vi "RTM CreateFramesSubSection.vi"(8 "error in (no error)":errorcluster, 11 "Node Ptr":T1 format="%.0x") -> (0 "error out":errorcluster, 3 "Node Ptr 2":T1 format="%.0x")   [LabVIEW 2018, in "CAN Gateway System Explorer.lvlib"]
uses:
  CAN Gateway System Explorer.lvlib
  <vilib>/NI Veristand/Custom Device API/Custom Device Item Ref.ctl
  <vilib>/NI Veristand/Custom Device API/Custom Device Channel.ctl
  <vilib>/NI Veristand/Custom Device API/Custom Device Channel Type.ctl
  Shared/Constants.vi
  <vilib>/NI Veristand/Custom Device API/Custom Device API.lvlib
  Shared/CAN Gateway Shared.lvlib
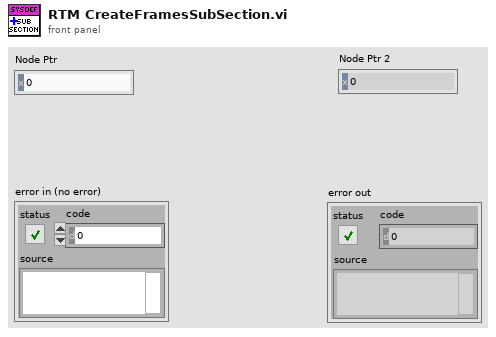
[diagram p1: front panel]
types:
  T1 = typedef "Custom Device API.lvlib/Custom Device Item Ref.ctl" = u64
  T2 = typedef "Custom Device API.lvlib/Custom Device Channel.ctl" = cluster{"Type":T3, "Units":string, "Default Value":dbl, "Faultable":bool, "Scalable":bool}
  T3 = typedef "Custom Device API.lvlib/Custom Device Channel Type.ctl" = enum16{"Input", "Output"}
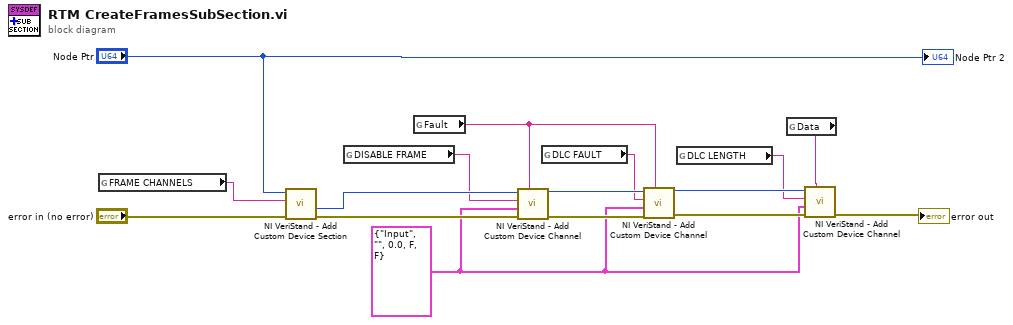
[diagram p0: block diagram]
diagram:
  w4 = T2 {"Type"=enum."Input", "Units"="", "Default Value"=0.0, "Faultable"=FALSE, "Scalable"=FALSE} ("Channel")
  n1 = global read "Constants.vi" "FRAME CHANNELS"() -> (w14:string)
  n2 = call <vilib>:"NI VeriStand - Add Custom Device Section.vi"("error in (no error)"="error in (no error)", "Section Name"=w14, "Parent Ref in"="Node Ptr") -> ("error out"=w12:errorcluster, "Section Ptr"=w13:T1)  [unwired: 5 in, 2 out]
  n3 = global read "Constants.vi" "DISABLE FRAME"() -> (w11:string)
  n4 = global read "Constants.vi" "Fault"() -> (w3:string)
  n5 = call <vilib>:"NI VeriStand - Add Custom Device Channel.vi"("GUID (Default Channel)"=w3, "error in (no error)"=w12, "Channel"=w4, "Channel Name"=w11, "Parent Ref in"=w13) -> ("error out"=w8:errorcluster, "Parent Ref out"=w10:T1)  [unwired: 3 in, 2 out]
  n6 = global read "Constants.vi" "DLC FAULT"() -> (w9:string)
  n7 = call <vilib>:"NI VeriStand - Add Custom Device Channel.vi"("GUID (Default Channel)"=w3, "error in (no error)"=w8, "Channel"=w4, "Channel Name"=w9, "Parent Ref in"=w10) -> ("error out"=w7:errorcluster, "Parent Ref out"=w6:T1)  [unwired: 3 in, 2 out]
  n8 = global read "Constants.vi" "DLC LENGTH"() -> (w5:string)
  n9 = global read "Constants.vi" "Data"() -> (w2:string)
  n10 = call <vilib>:"NI VeriStand - Add Custom Device Channel.vi"("GUID (Default Channel)"=w2, "error in (no error)"=w7, "Channel"=w4, "Channel Name"=w5, "Parent Ref in"=w6) -> ("error out"=→"error out":errorcluster)  [unwired: 3 in, 3 out]
  "Node Ptr 2" <- "Node Ptr"
